vi "opencvSegmentConvertCoordinates-singleFrame.vi"(1 "sizex2":u16=256, 2 "NeuronN":u16, 3 "NeuronXY":u16[](array[numeric])) -> (0 "XY":u16[][](array[numeric]))   [LabVIEW 2017]
panel:
  # "XY[coordinate,neuron]"
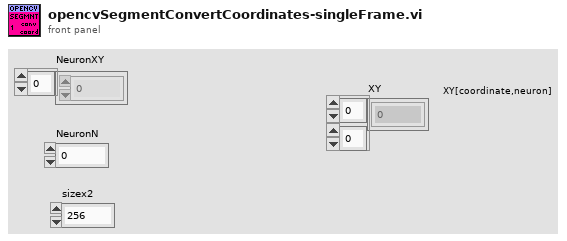
[diagram p1: front panel]
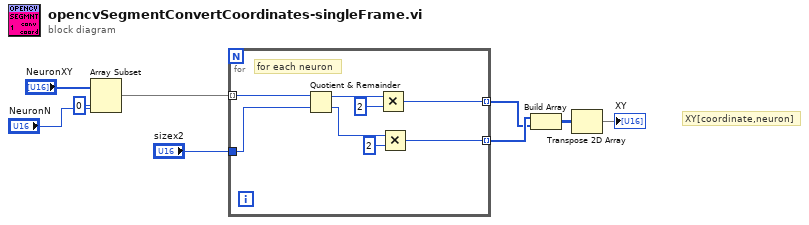
[diagram p0: block diagram]
diagram:
  # "XY[coordinate,neuron]"
  n1 = Array Subset(array="NeuronXY", index=0, length="NeuronN") -> (w3:u16[])
  n2 = for {
    tunnel: w3 -> [w13] mode=indexing
    tunnel: "sizex2" -> [w12]
    tunnel: [w11] -> w1 mode=indexing
    tunnel: [w10] -> w2 mode=indexing
    # "for each neuron"
    n3 = Quotient & Remainder(x=w13, y=w12) -> (x-y*floor(x/y)=w16:u16, floor(x/y)=w17:u16)
    n4 = Multiply(x=w16, y=u16 2) -> (x*y=w11:u16)
    n5 = Multiply(x=w17, y=u16 2) -> (x*y=w10:u16)
  }
  n6 = Build Array(w2, w1) -> (w8:u16[][])
  n7 = Transpose 2D Array(2D array=w8) -> (transposed array=→"XY":u16[][])
